vi "Queue Obtain.vi"() -> (0 "error out":errorcluster, 2 "Queue":refnum<data-value>)   [LabVIEW 2021, in "jettl Queue Actor.lvlib"]
uses:
  jettl Queue Actor.lvlib
  Actor/Msg/Msg.lvclass
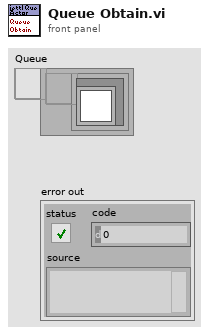
[diagram p1: front panel]
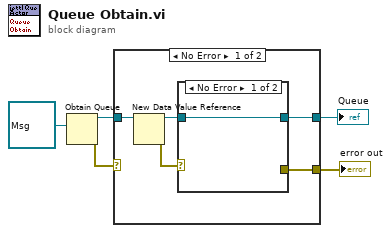
[diagram p0: block diagram]
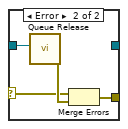
[diagram p2: hidden frame]
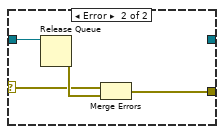
[diagram p3: hidden frame]
diagram:
  n1 = Obtain Queue(element data type=refnum<class "Msg.lvclass"> refnum ("Msg.lvclass")) -> (queue out=w4:refnum<queue>, error out=w5:errorcluster)  [unwired: 4 in, 1 out]
  n2 = case shown="No Error" w5 {
    selector: w5 -> [_ w16]
    tunnel: w4 -> [w10 w19]
    tunnel: [w7 _] -> w1
    tunnel: [w8 w18] -> w3
    frame No Error {
      n3 = New Data Value Reference(data value=w10) -> (data value reference=w6:refnum<data-value>, error out=w9:errorcluster)  [unwired: 1 in]
      n4 = case shown="No Error" w9 {
        selector: w9 -> [_ w12]
        tunnel: [_ w14] -> w8
        tunnel: [w11 _] -> w7
        tunnel: w6 -> [w11 w15]
        frame No Error {
        }
        frame Error {
          n5 = call "Queue Release.vi"("Queue"=w15) -> ("error out"=w13:errorcluster)  [unwired: 10 in]
          n6 = Merge Errors(w12, w13) -> (w14:errorcluster)
        }
      }
    }
    frame Error {
      n7 = Release Queue(queue=w19) -> (error out=w17:errorcluster)  [unwired: 2 in, 2 out]
      n8 = Merge Errors(w16, w17) -> (w18:errorcluster)
    }
  }
  "error out" <- w3
  "Queue" <- w1
